vi "WalkaboutRepository.vi"(0 "reference in":refnum<class "Object.lvclass">, 1 "Action(ReadRepository)":T1(ring), 5 "error in (no error)":errorcluster) -> (9 "ProcessViRef":refnum<vi>, 11 "ProcessSyncOccurrence":refnum<k4>, 13 "FromProcessQueue":refnum<queue>, 14 "reference out":refnum<class "Object.lvclass">, 15 "ToProcessQueue":refnum<queue>, 17 "ProcessAlreadyStarted":bool, 19 "error out":errorcluster)   [LabVIEW 2019, in "Object.lvclass"]
uses:
  Object.lvclass
  Walkabout.ctl
  Object.lvclass/Object.ctl
panel:
  # "Use this indicator for sending messages to the Process VI"
  # "These indicators are used by the process VIs"
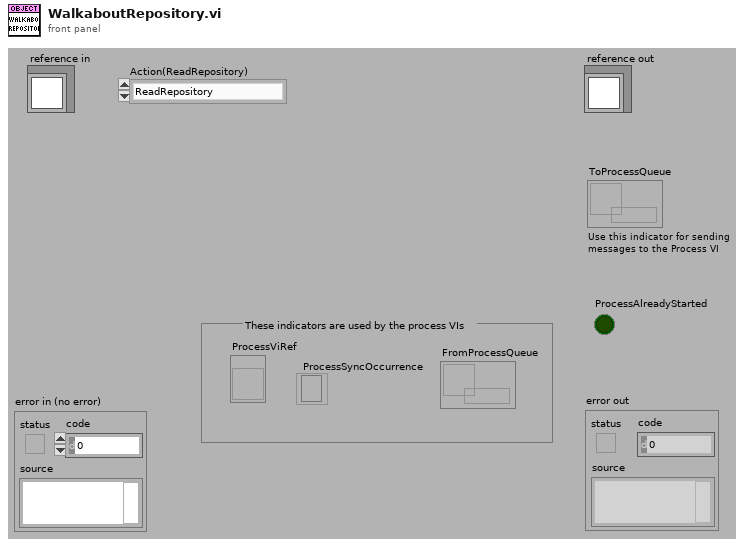
[diagram p1: front panel]
types:
  T1 = enum16{"ReadRepository", "CreateNew", "CreateOrLookUpExisting"}
  T2 = typedef "Object.lvclass/Walkabout.ctl" = cluster{"ToProcessQueue":refnum<queue>, "FromProcessQueue":refnum<queue>, "ProcessSyncOccurrence":refnum<k4>, "ProcessViRef":refnum<vi>}
  T3 = typedef "Object.lvclass/ObjectReference.ctl" = refnum<k1>
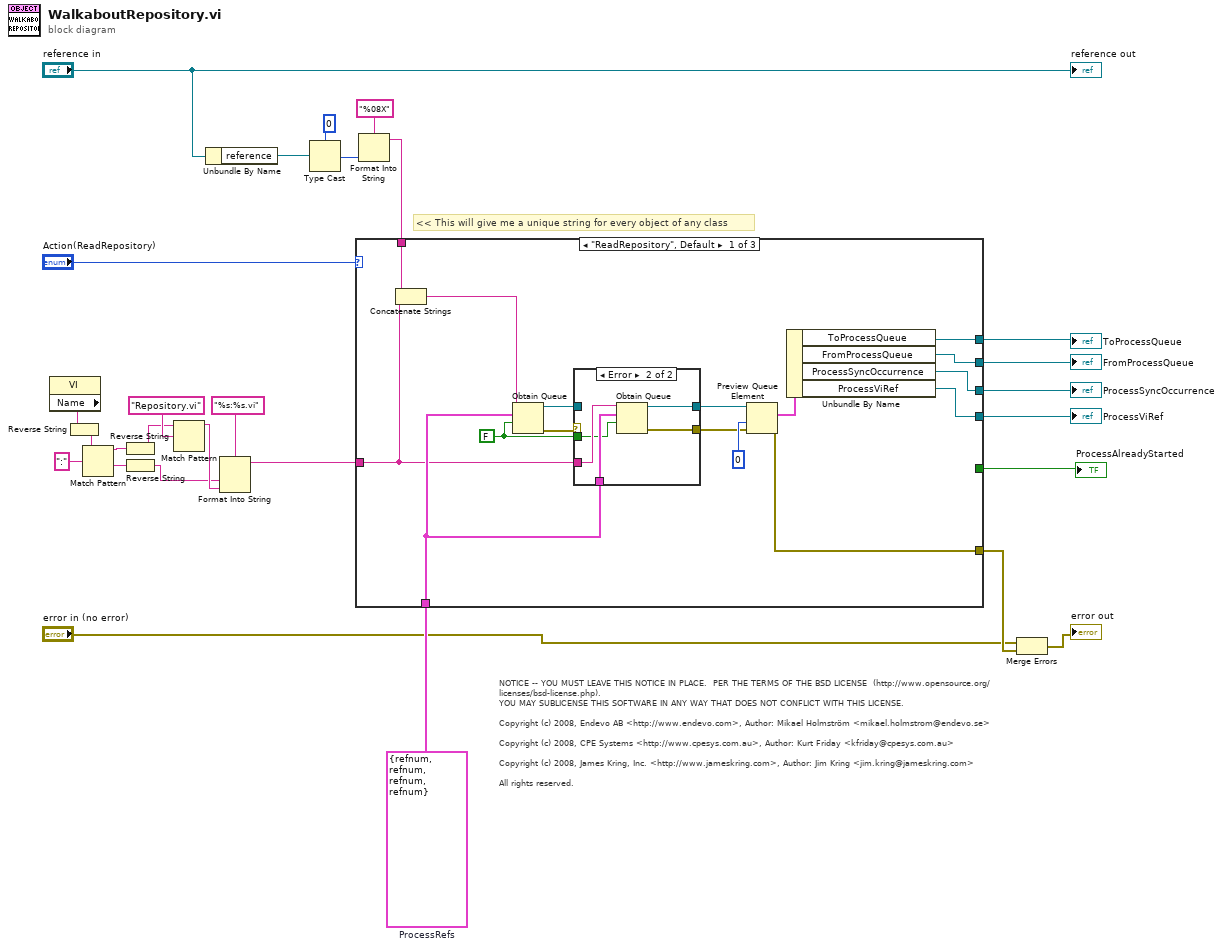
[diagram p0: block diagram]
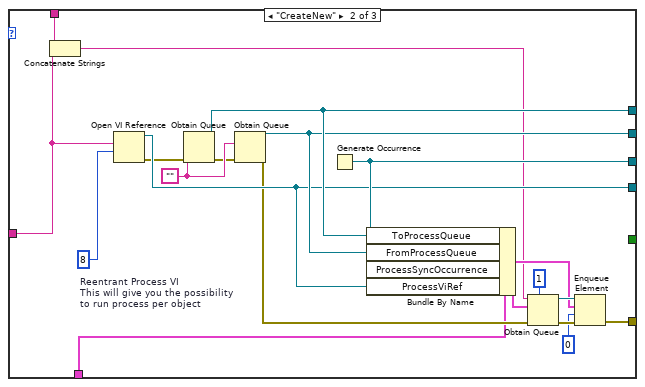
[diagram p3: hidden frame]
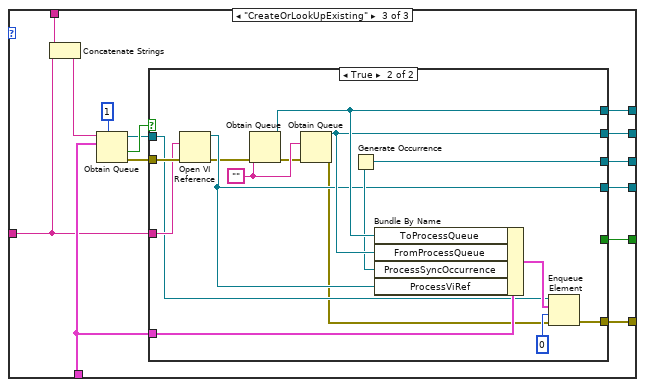
[diagram p4: hidden frame]
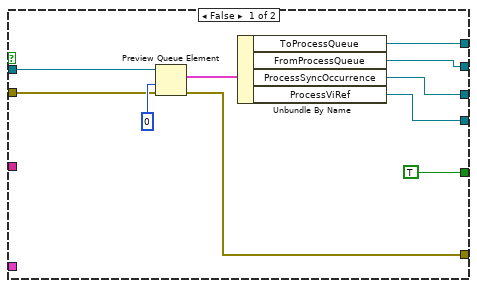
[diagram p5: hidden frame]
diagram:
  w22 = T2 {"ToProcessQueue"=refnum, "FromProcessQueue"=refnum, "ProcessSyncOccurrence"=refnum, "ProcessViRef"=refnum}  # ProcessRefs
  # "NOTICE -- YOU MUST LEAVE THIS NOTICE IN PLACE.  PER THE TERMS OF THE BSD LICENSE  (http://www.opensource.org/licenses/bsd-license.php).\nYOU MAY SUBLICENSE THIS SOFTWARE IN ANY WAY THAT DOES NOT CONFLICT WITH THIS LICENSE.\n\nCopyright (c) 2008, Endevo AB <http://www.endevo.com>, Author: Mikael Holmström <mikael.holmstrom@endevo.se>\n\nCopyright (c) 2008, CPE Systems <http://www.cpesys.com.au>, Author: Kurt Friday <kfriday@cpesys.com.au>\n\nCopyright (c) 2008, James Kring, Inc. <http://www.jameskring.com>, Author: Jim Kring <jim.kring@jameskring.com>\n\nAll rights reserved."
  # "<< This will give me a unique string for every object of any class"
  n1 = property class="VI"() -> ("Name"=w11:string)  [unwired: 2 in, 2 out]
  n2 = Reverse String(1:w11) -> (0:w12:string)
  n3 = Match Pattern(string=w12, regular expression=":") -> (before substring=w16:string, after substring=w13:string)  [unwired: 3 out]
  n4 = Reverse String(1:w16) -> (0:w17:string)
  n5 = Reverse String(1:w13) -> (0:w15:string)
  n6 = Match Pattern(string=w17, regular expression="Repository.vi") -> (before substring=w19:string)  [unwired: 4 out]
  n7 = Unbundle By Name("reference in") -> ("reference"=w1:T3)
  n8 = Format Into String(format string="%s:%s.vi", w15, w19) -> (resulting string=w9:string)  [unwired: 2 in, 1 out]
  n9 = Type Cast(type=u32 0, x=w1) -> (*(type *) &x=w6:u32)
  n10 = Format Into String(format string="%08X", w6) -> (resulting string=w3:string)  [unwired: 2 in, 1 out]
  n11 = case shown="\"ReadRepository\", Default" "Action(ReadRepository)" {
    tunnel: [w38 w67 w81] -> w26
    tunnel: [w40 w69 w83] -> w24
    tunnel: [w39 w68 w82] -> w25
    tunnel: [w41 w66 w80] -> w23
    tunnel: w22 -> [w32 w54 w76]
    tunnel: w3 -> [w30 w53 w72]
    tunnel: [w37 w65 w79] -> w20
    tunnel: w9 -> [w29 w51 w71]
    tunnel: [_ _ w74] -> w8
    frame "ReadRepository", Default {
      w31 = FALSE ("create if not found? (T)")
      n12 = Concatenate Strings(w30, w29) -> (w28:string)
      n13 = Obtain Queue(name (unnamed)=w28, element data type=w32, create if not found? (T)=w31) -> (queue out=w34:refnum<queue>, error out=w36:errorcluster)  [unwired: 2 in, 1 out]
      n14 = case shown="Error" w36 {
        selector: w36 -> [w45 _]
        tunnel: [w45 w47] -> w35
        tunnel: w34 -> [w44 _]
        tunnel: [w44 w48] -> w33
        tunnel: w32 -> [_ w50]
        tunnel: w29 -> [_ w49]
        tunnel: w31 -> [_ w46]
        frame No Error {
        }
        frame Error {
          n15 = Obtain Queue(name (unnamed)=w49, element data type=w50, create if not found? (T)=w46) -> (queue out=w48:refnum<queue>, error out=w47:errorcluster)  [unwired: 2 in, 1 out]
        }
      }
      n16 = Preview Queue Element(queue=w33, timeout in ms (-1)=0, error in (no error)=w35) -> (element=w42:T2, error out=w37:errorcluster)  [unwired: 2 out]
      n17 = Unbundle By Name(w42) -> ("ToProcessQueue"=w40:refnum<queue>, "FromProcessQueue"=w39:refnum<queue>, "ProcessSyncOccurrence"=w38:refnum<k4>, "ProcessViRef"=w41:refnum<vi>)
    }
    frame "CreateNew" {
      w61 = 8  # Reentrant Process VI This will give you the possibility to run process per object
      w64 = ""
      n18 = Concatenate Strings(w53, w51) -> (w52:string)
      n19 = Open VI Reference(vi path=w51, options=w61) -> (vi reference=w66:refnum<vi>, error out=w62:errorcluster)  [unwired: 1 in, 3 out]
      n20 = Obtain Queue(element data type=w64, error in (no error)=w62) -> (queue out=w69:refnum<queue>, error out=w63:errorcluster)  [unwired: 2 in, 2 out]
      n21 = Obtain Queue(element data type=w64, error in (no error)=w63) -> (queue out=w68:refnum<queue>, error out=w56:errorcluster)  [unwired: 2 in, 2 out]
      n22 = Generate Occurrence() -> (w67:refnum<k4>)
      n23 = Bundle By Name(cluster=w54, "ToProcessQueue"=w69, "FromProcessQueue"=w68, "ProcessSyncOccurrence"=w67, "ProcessViRef"=w66) -> (w58:T2)
      n24 = Obtain Queue(max queue size (-1, unlimited)=1, name (unnamed)=w52, element data type=w58, error in (no error)=w56) -> (queue out=w60:refnum<queue>, error out=w59:errorcluster)  [unwired: 1 in, 1 out]
      n25 = Enqueue Element(queue=w60, element=w58, timeout in ms (-1)=0, error in (no error)=w59) -> (error out=w65:errorcluster)  [unwired: 2 out]
    }
    frame "CreateOrLookUpExisting" {
      n26 = Concatenate Strings(w72, w71) -> (w70:string)
      n27 = Obtain Queue(max queue size (-1, unlimited)=1, name (unnamed)=w70, element data type=w76) -> (queue out=w77:refnum<queue>, created new?=w78:bool, error out=w75:errorcluster)  [unwired: 2 in]
      n28 = case shown="True" w78 {
        tunnel: [w93 w108] -> w83
        tunnel: [w92 w107] -> w82
        tunnel: [w91 w106] -> w81
        tunnel: [w90 w105] -> w80
        tunnel: [w86 w104] -> w79
        tunnel: w76 -> [_ w103]
        tunnel: w75 -> [w87 w97]
        tunnel: w71 -> [_ w96]
        tunnel: w77 -> [w88 w95]
        tunnel: [TRUE _] -> w74
        frame False {
          n29 = Preview Queue Element(queue=w88, timeout in ms (-1)=0, error in (no error)=w87) -> (element=w85:T2, error out=w86:errorcluster)  [unwired: 2 out]
          n30 = Unbundle By Name(w85) -> ("ToProcessQueue"=w93:refnum<queue>, "FromProcessQueue"=w92:refnum<queue>, "ProcessSyncOccurrence"=w91:refnum<k4>, "ProcessViRef"=w90:refnum<vi>)
        }
        frame True {
          w102 = ""
          n31 = Open VI Reference(vi path=w96, error in (no error)=w97) -> (vi reference=w105:refnum<vi>, error out=w100:errorcluster)  [unwired: 4 out]
          n32 = Obtain Queue(element data type=w102, error in (no error)=w100) -> (queue out=w108:refnum<queue>, error out=w101:errorcluster)  [unwired: 2 in, 2 out]
          n33 = Obtain Queue(element data type=w102, error in (no error)=w101) -> (queue out=w107:refnum<queue>, error out=w94:errorcluster)  [unwired: 2 in, 2 out]
          n34 = Generate Occurrence() -> (w106:refnum<k4>)
          n35 = Bundle By Name(cluster=w103, "ToProcessQueue"=w108, "FromProcessQueue"=w107, "ProcessSyncOccurrence"=w106, "ProcessViRef"=w105) -> (w99:T2)
          n36 = Enqueue Element(queue=w95, element=w99, timeout in ms (-1)=0, error in (no error)=w94) -> (error out=w104:errorcluster)  [unwired: 2 out]
        }
      }
    }
  }
  "ProcessSyncOccurrence" <- w26
  "ToProcessQueue" <- w24
  "FromProcessQueue" <- w25
  "ProcessViRef" <- w23
  "ProcessAlreadyStarted" <- w8
  n37 = Merge Errors("error in (no error)", w20) -> (→"error out":errorcluster)
  "reference out" <- "reference in"
